vi "Copy Builds To NIVS Dir.vi"(5 "Files Generated by Build":path[](array[path]), 6 "Top Level/Always Included VIs":path[](array[path]), 7 "Destination Path":path, 8 "error in (no error)":errorcluster, 9 "Target Name":string, 10 "Build Specification Name":string, 11 "Project Path":path) -> (0 "error out":errorcluster)   [LabVIEW 2026]
uses:
  C:/Users/ppathak/Downloads/NationalInstruments.VeriStand.dll
  Users/ppathak/Downloads/NationalInstruments.VeriStand.dll
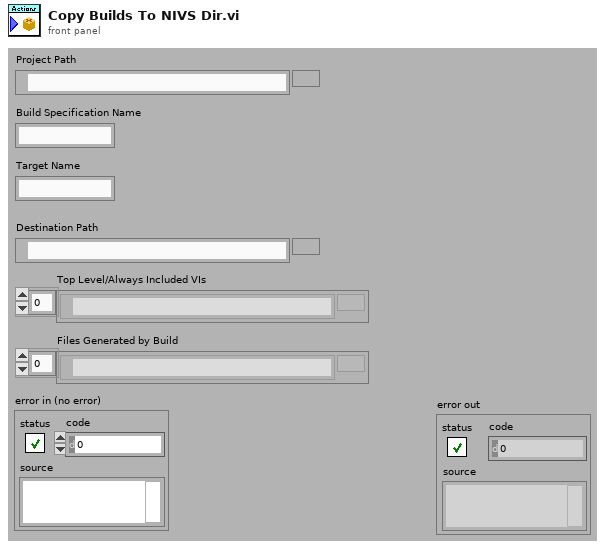
[diagram p1: front panel]
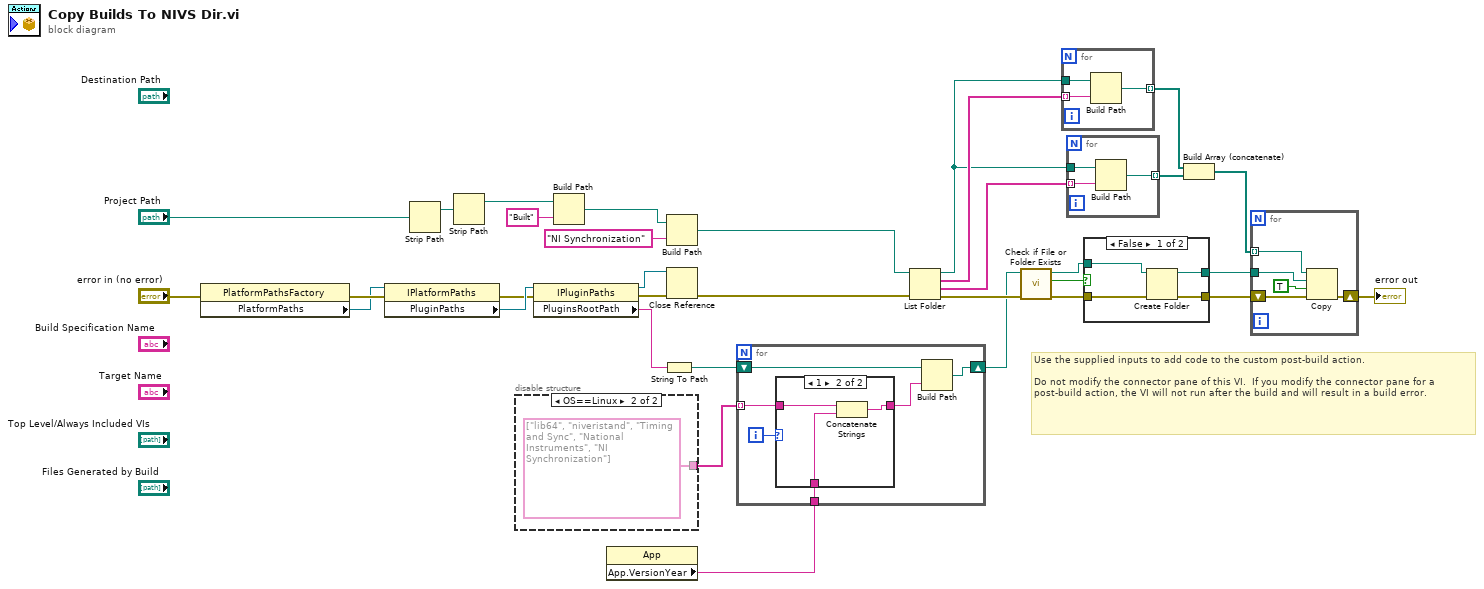
[diagram p0: block diagram]
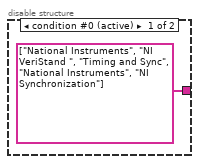
[diagram p3: hidden frame]
diagram:
  # "Use the supplied inputs to add code to the custom post-build action.\n\nDo not modify the connector pane of this VI.  If you modify the connector pane for a post-build action, the VI will not run after the build and will result in a build error."
  n1 = property class="PlatformPathsFactory"(error in="error in (no error)") -> (error out=w9:errorcluster, "PlatformPaths"=w7:refnum<k24>)  [unwired: 1 in, 1 out]
  n2 = property class="IPlatformPaths"(reference=w7, error in=w9) -> (error out=w8:errorcluster, "PluginPaths"=w10:refnum<k24>)  [unwired: 1 out]
  n3 = Strip Path(path="Project Path") -> (stripped path=w18:path)  [unwired: 1 out]
  n4 = Strip Path(path=w18) -> (stripped path=w29:path)  [unwired: 1 out]
  n5 = disable-structure shown="OS==Linux" {
    disable-tunnel: [string[] ["National Instruments", "NI VeriStand ", "Timing and Sync", "National Instruments", "NI Synchronization"] string[] ["lib64", "niveristand", "Timing and Sync", "National Instruments", "NI Synchronization"]] -> w15
    frame condition #0 (active) {
    }
    frame condition #1 {
    }
  }
  n6 = property class="IPluginPaths"(reference=w10, error in=w8) -> (reference out=w1:refnum<k24>, error out=w5:errorcluster, "PluginsRootPath"=w6:string)
  n7 = Build Path(base path=w29, name or relative path="Built") -> (appended path=w12:path)
  n8 = property class="App"() -> ("App.VersionYear"=w13:string)  [unwired: 2 in, 2 out]
  n9 = String To Path(string=w6) -> (path=w3:path)
  n10 = Build Path(base path=w12, name or relative path="NI Synchronization") -> (appended path=w17:path)
  n11 = Close Reference(reference=w1, error in (no error)=w5) -> (error out=w2:errorcluster)
  n12 = for {
    shift-right: [w40] -> w14
    shift-left: w3 -> [w41]
    tunnel: w15 -> [w37] mode=indexing
    tunnel: w13 -> [w36]
    i -> [w39]
    n13 = case shown="1" w39 {
      tunnel: [w42 w44] -> w38
      tunnel: w37 -> [w42 w45]
      tunnel: w36 -> [_ w43]
      frame Default {
      }
      frame 1 {
        n14 = Concatenate Strings(w45, w43) -> (w44:string)
      }
    }
    n15 = Build Path(base path=w41, name or relative path=w38) -> (appended path=w40:path)
  }
  n16 = List Folder(path=w17, error in=w2) -> (path out=w20:path, filenames=w33:string[], folder names=w21:string[], error out=w16:errorcluster)  [unwired: 2 in]
  n17 = call <vilib>:"Check if File or Folder Exists.vi"("error in (no error)"=w16, "path"=w14) -> ("error out"=w24:errorcluster, "file or folder exists?"=w26:bool, "dup path"=w25:path)  [unwired: 7 in]
  n18 = for {
    tunnel: w33 -> [w47] mode=indexing
    tunnel: w20 -> [w48]
    tunnel: [w46] -> w32 mode=indexing
    n19 = Build Path(base path=w48, name or relative path=w47) -> (appended path=w46:path)
  }
  n20 = for {
    tunnel: w21 -> [w50] mode=indexing
    tunnel: w20 -> [w51]
    tunnel: [w49] -> w19 mode=indexing
    n21 = Build Path(base path=w51, name or relative path=w50) -> (appended path=w49:path)
  }
  n22 = case shown="False" w26 {
    tunnel: w25 -> [w55 w57]
    tunnel: w24 -> [w54 w56]
    tunnel: [w53 w57] -> w23
    tunnel: [w52 w56] -> w22
    frame False {
      n23 = Create Folder(path (use dialog)=w55, error in=w54) -> (created path=w53:path, error out=w52:errorcluster)  [unwired: 1 in, 1 out]
    }
    frame True {
    }
  }
  n24 = Build Array (concatenate)(w32, w19) -> (w31:path[])
  n25 = for {
    tunnel: w31 -> [w59] mode=indexing
    shift-right: [w60] -> w11
    shift-left: w22 -> [w61]
    tunnel: w23 -> [w58]
    n26 = Copy(8:w61, 9:TRUE ("overwrite (F)"), 10:w58, 11:w59) -> (0:w60:errorcluster)  [unwired: 1 in, 2 out]
  }
  "error out" <- w11
